vi "calibrate range.vi"   [LabVIEW 2016, in "Test2.lvrbt"]
uses:
  Test2.lvrbt
  <vilib>/NXT/Block Support/NXT_InputPort.ctl
  <vilib>/NXT/Hardware/Plugins/Tetrix DC Motor/TetrixDCMotorAddress.ctl
  <vilib>/NXT/NXTIO Xnodes/NXTIONodeSubVIs/TETRIX IO Move DC Motors.vi
  <vilib>/NXT/Dual Mode Library/Waits/Wait_EV3_Ultrasonic_Centimeter_Closer.vi
  <vilib>/NXT/NXTIO Xnodes/NXTIONodeSubVIs/TETRIX IO Stop DC Motors.vi
  <vilib>/NXT/Dual Mode Library/Waits/Wait_Num.vi
  <vilib>/NXT/Dual Mode Library/Waits/Wait_EV3_Ultrasonic_Centimeters_Further.vi
  <vilib>/NXT/Subs/LVHSConnector.ctl
  <vilib>/NXT/NXTIO Xnodes/AddressXNode/NXTIOAddress.xnode
  <vilib>/NXT/NXTIO Xnodes/NXTIOXNode/NXTIO.xnode
  <vilib>/NXT/LegoClasses/BrickReference/BrickReference.lvclass
types:
  T1 = typedef "NXT_InputPort.ctl" = u32
  T2 = typedef "TetrixDCMotorAddress.ctl" = i32
  T3 = typedef "LVHSConnector.ctl" = refnum<class "BrickReference.lvclass">
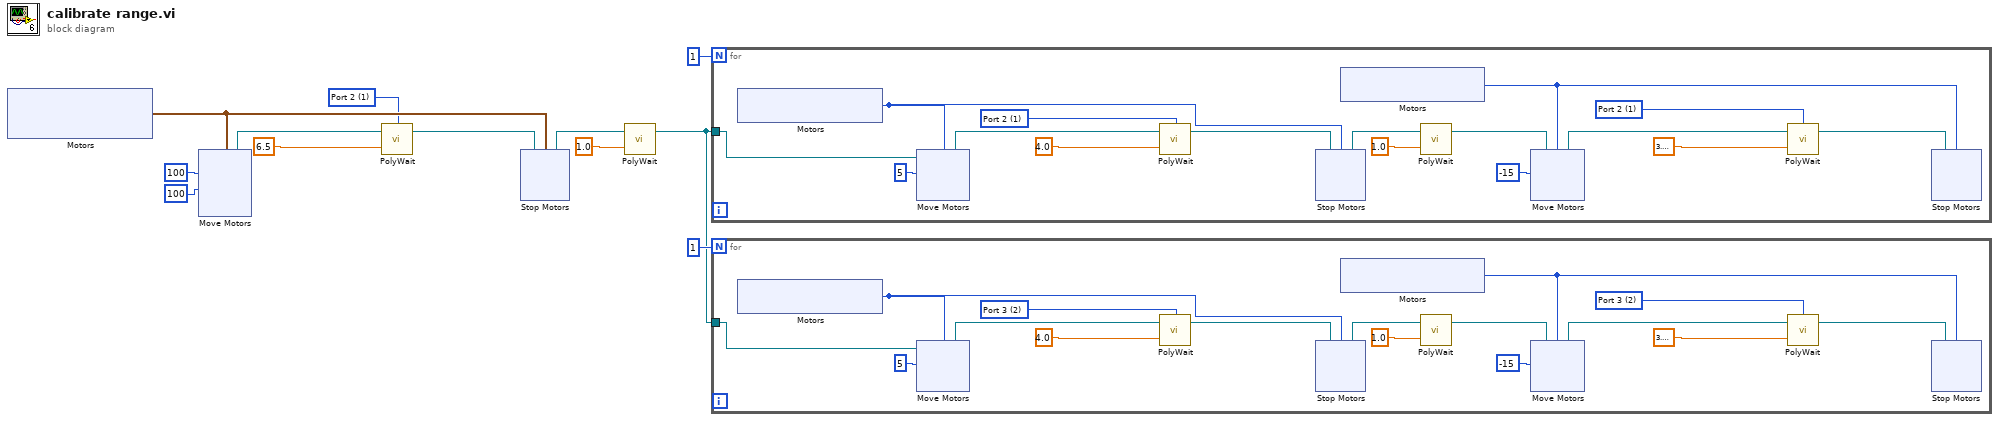
[diagram p0: block diagram]
diagram:
  w1 = T1 1 items=["Port 1", "Port 2", "Port 3", "Port 4"] ("Port (Port 1)")
  n1 = xnode "Motors"() -> ("Motor"=w7:cluster{"TetrixDCMotor":T2, "TetrixDCMotor":T2})
  n2 = xnode "Move Motors"("Power/Speed 2"=i8 100, "Power/Speed 1"=i8 100, "Motors"=w7) -> ("NXT/EV3"=w10:T3)  [unwired: 1 in]
  n3 = call-poly <vilib>:"PolyWait.vi"("Centimeters (40)"=sgl 6.5, "NXT/EV3"=w10, "Port (Port 1)"=w1) -> ("NXT/EV3"=w8:T3)  [unwired: 1 in]
  n4 = xnode "Stop Motors"("Motors"=w7, "NXT/EV3"=w8) -> ("NXT/EV3"=w4:T3)
  n5 = call-poly <vilib>:"PolyWait.vi"("Time (1 sec)"=sgl 1.0, "NXT/EV3"=w4) -> ("NXT/EV3"=w2:T3)  [unwired: 2 in]
  n6 = for {
    N: 1 -> [_]
    tunnel: w2 -> [w13]
    w17 = T1 1 items=["Port 1", "Port 2", "Port 3", "Port 4"] ("Port (Port 1)")
    w18 = T1 1 items=["Port 1", "Port 2", "Port 3", "Port 4"] ("Port (Port 1)")
    n7 = xnode "Motors"() -> ("Motor"=w24:T2)
    n8 = xnode "Move Motors"("Power/Speed 1"=i8 5, "Motors"=w24, "NXT/EV3"=w13) -> ("NXT/EV3"=w27:T3)
    n9 = call-poly <vilib>:"PolyWait.vi"("Centimeters (40)"=sgl 4.0, "NXT/EV3"=w27, "Port (Port 1)"=w18) -> ("NXT/EV3"=w25:T3)  [unwired: 1 in]
    n10 = xnode "Stop Motors"("Motors"=w24, "NXT/EV3"=w25) -> ("NXT/EV3"=w22:T3)
    n11 = xnode "Motors"() -> ("Motor"=w14:T2)
    n12 = call-poly <vilib>:"PolyWait.vi"("Time (1 sec)"=sgl 1.0, "NXT/EV3"=w22) -> ("NXT/EV3"=w21:T3)  [unwired: 2 in]
    n13 = xnode "Move Motors"("Power/Speed 1"=i8 -15, "Motors"=w14, "NXT/EV3"=w21) -> ("NXT/EV3"=w19:T3)
    n14 = call-poly <vilib>:"PolyWait.vi"("Centimeters (50)"=sgl 3.2, "NXT/EV3"=w19, "Port (Port 1)"=w17) -> ("NXT/EV3"=w15:T3)  [unwired: 1 in]
    n15 = xnode "Stop Motors"("Motors"=w14, "NXT/EV3"=w15) -> ()  [unwired: 1 out]
  }
  n16 = for {
    N: 1 -> [_]
    tunnel: w2 -> [w55]
    w60 = T1 2 items=["Port 1", "Port 2", "Port 3", "Port 4"] ("Port (Port 1)")
    w61 = T1 2 items=["Port 1", "Port 2", "Port 3", "Port 4"] ("Port (Port 1)")
    n17 = xnode "Motors"() -> ("Motor"=w59:T2)
    n18 = xnode "Move Motors"("Power/Speed 1"=i8 5, "Motors"=w59, "NXT/EV3"=w55) -> ("NXT/EV3"=w69:T3)
    n19 = call-poly <vilib>:"PolyWait.vi"("Centimeters (40)"=sgl 4.0, "NXT/EV3"=w69, "Port (Port 1)"=w61) -> ("NXT/EV3"=w67:T3)  [unwired: 1 in]
    n20 = xnode "Stop Motors"("Motors"=w59, "NXT/EV3"=w67) -> ("NXT/EV3"=w65:T3)
    n21 = xnode "Motors"() -> ("Motor"=w57:T2)
    n22 = call-poly <vilib>:"PolyWait.vi"("Time (1 sec)"=sgl 1.0, "NXT/EV3"=w65) -> ("NXT/EV3"=w64:T3)  [unwired: 2 in]
    n23 = xnode "Move Motors"("Power/Speed 1"=i8 -15, "Motors"=w57, "NXT/EV3"=w64) -> ("NXT/EV3"=w62:T3)
    n24 = call-poly <vilib>:"PolyWait.vi"("Centimeters (50)"=sgl 3.2, "NXT/EV3"=w62, "Port (Port 1)"=w60) -> ("NXT/EV3"=w56:T3)  [unwired: 1 in]
    n25 = xnode "Stop Motors"("Motors"=w57, "NXT/EV3"=w56) -> ()  [unwired: 1 out]
  }
